vi "unit_tester.vi"() -> ()   [LabVIEW 2020]
panel:
  out "Array":cluster{"expression out":string, bool}[](array[cluster])
  in  "Test files":T1(array[cluster])=[{"input_lablisp_file"=path "/Users/joris/repos/labview_lisp/test/cylinder-volume.lablisp", "expected_equivalent_output"=path "/Users/joris/repos/labview_lisp/test/cylinder-volume_expected.lablisp"}, {"input_lablisp_file"=path "/Users/joris/repos/labview_lisp/test/define-tau.lablisp", "expected_equivalent_output"=path "/Users/joris/repos/labview_lisp/test/define-tau_expected.lablisp"}, {"input_lablisp_file"=path "/Users/joris/repos/labview_lisp/test/factorial.lablisp", "expected_equivalent_output"=path "/Users/joris/repos/labview_lisp/test/factorial_expected.lablisp"}, {"input_lablisp_file"=path "/Users/joris/repos/labview_lisp/test/and.lablisp", "expected_equivalent_output"=path "/Users/joris/repos/labview_lisp/test/and_expected.lablisp"}, {"input_lablisp_file"=path "/Users/joris/repos/labview_lisp/test/or.lablisp ", "expected_equivalent_output"=path "/Users/joris/repos/labview_lisp/test/or_expected.lablisp "}, {"input_lablisp_file"=path "/Users/joris/repos/labview_lisp/test/let.lablisp ", "expected_equivalent_output"=path "/Users/joris/repos/labview_lisp/test/let_expected.lablisp"}, {"input_lablisp_file"=path "/Users/joris/repos/labview_lisp/test/cond.lablisp", "expected_equivalent_output"=path "/Users/joris/repos/labview_lisp/test/cond_expected.lablisp"}, {"input_lablisp_file"=path "/Users/joris/repos/labview_lisp/test/fibonacci.lablisp", "expected_equivalent_output"=path "/Users/joris/repos/labview_lisp/test/fibonacci_expected.lablisp"}, {"input_lablisp_file"=path "/Users/joris/repos/labview_lisp/test/number_test.lablisp", "expected_equivalent_output"=path "/Users/joris/repos/labview_lisp/test/number_test_expected.lablisp"}]
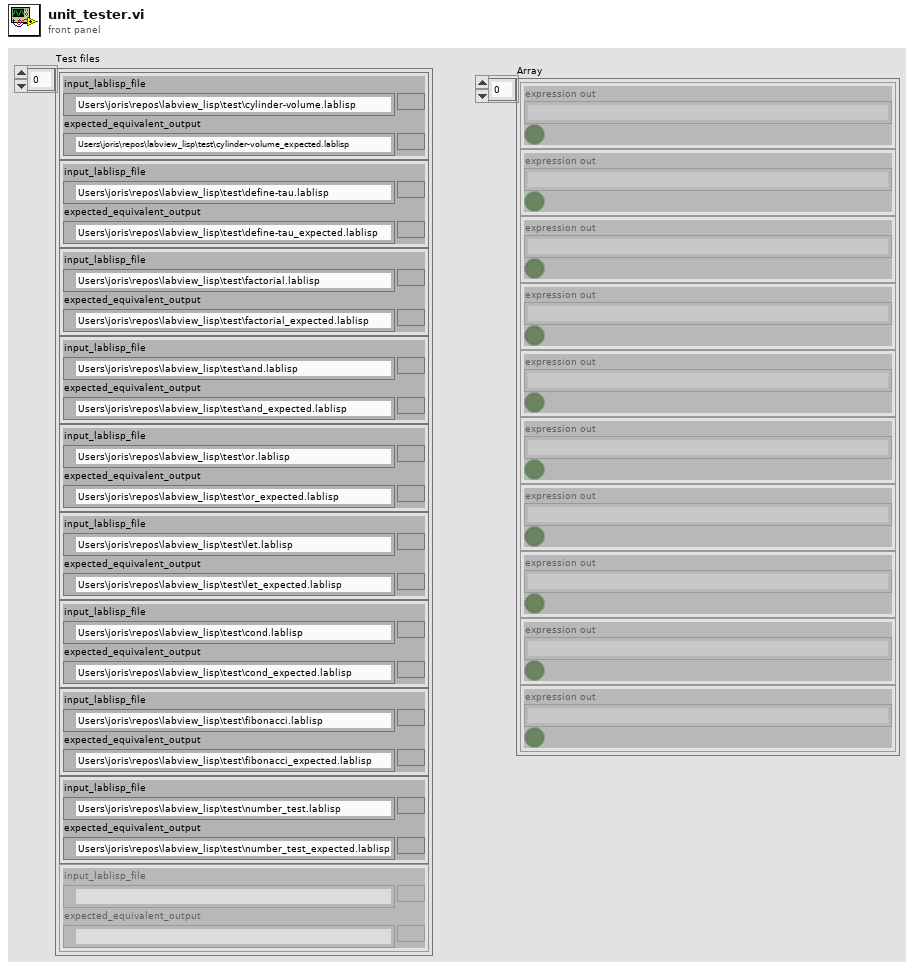
[diagram p1: front panel]
types:
  T1 = cluster{"input_lablisp_file":path, "expected_equivalent_output":path}[]
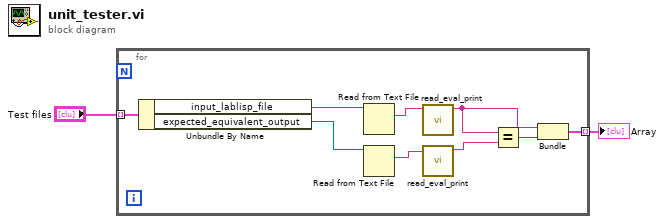
[diagram p0: block diagram]
diagram:
  n1 = for {
    tunnel: "Test files" -> [w11] mode=indexing
    tunnel: [w3] -> w1 mode=indexing
    n2 = Unbundle By Name(w11) -> ("input_lablisp_file"=w10:path, "expected_equivalent_output"=w9:path)
    n3 = Read from Text File(file (use dialog)=w10) -> (text=w8:string)  [unwired: 3 in, 3 out]
    n4 = Read from Text File(file (use dialog)=w9) -> (text=w7:string)  [unwired: 3 in, 3 out]
    n5 = call "read_eval_print.vi"("input string"=w8) -> ("expression out"=w4:string)  [unwired: 9 in, 1 out]
    n6 = call "read_eval_print.vi"("input string"=w7) -> ("expression out"=w6:string)  [unwired: 9 in, 1 out]
    n7 = Equal?(x=w4, y=w6) -> (x = y?=w5:bool)
    n8 = Bundle("expression out"=w4, w5) -> (w3:cluster{"expression out":string, bool})  [unwired: 1 in]
  }
  "Array" <- w1
